vi "Configure Trigger (CAN - Start,EOF,Missing Ack).vi"(0 "VISA resource name":refnum<visa-resource-name>, 1 "Data Threshold (0.0V)":dbl, 2 "Nominal Bit Rate (1MB)":dbl=1000000.0, 3 "CAN Format (0:Standard)":u16(ring) items=["Standard", "Extended"], 5 "Source (0:Channel1)":u16(ring) items=["Channel1", "Channel2", "Channel3", "Channel4"], 7 "Signal Type (0:Differential)":u16(ring) items=["Differential", "CAN + H", "CAN - L", "TX", "RX"], 9 "Trigger Condition (0:Start)":u16(ring) items=["Start"=0, "EOF"=5, "Missing ack"=6], 11 "error in (no error)":errorcluster) -> (4 "VISA resource name out":refnum<visa-resource-name>, 15 "error out":errorcluster)   [LabVIEW 2015, in "Tektronix 7000 Series.lvlib"]
doc: "Configures CAN trigger settings(Start,EOF,Missing Ask) for an oscilloscope.A trigger occurs when a Controller Area Network frame signal is found.\n\n<b>Note:</b>\nOnly DPO7000 series oscilloscopes Support CAN Trigger."
uses:
  <instrlib>/Tektronix 7000 Series/Tektronix 7000 Series.lvlib
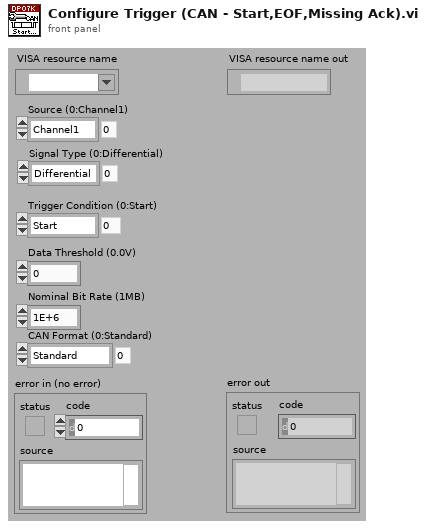
[diagram p1: front panel]
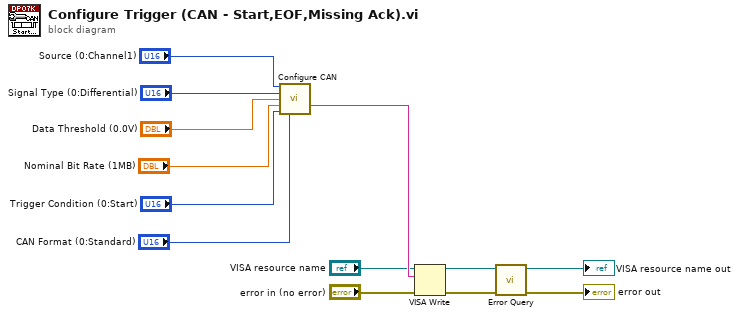
[diagram p0: block diagram]
diagram:
  n1 = call <instrlib>:"Configure CAN.vi"("Source (0:Channel1)"="Source (0:Channel1)", "Signal Type (0:Differential)"="Signal Type (0:Differential)", "Data Threshold (0.0V)"="Data Threshold (0.0V)", "Nominal Bit Rate (1MB)"="Nominal Bit Rate (1MB)", "Trigger Condition (0:Start)"="Trigger Condition (0:Start)", "CAN Format (0:Standard)"="CAN Format (0:Standard)") -> ("Output String"=w11:string)  [unwired: 9 in]
  n2 = VISA Write(VISA resource name="VISA resource name", write buffer=w11, error in (no error)="error in (no error)") -> (VISA resource name out=w12:refnum<visa-resource-name>, error out=w13:errorcluster)  [unwired: 1 out]
  n3 = call <instrlib>:"Error Query.vi"("error in (no error)"=w13, "VISA resource name"=w12) -> ("error out"=→"error out":errorcluster, "VISA resource name out"=→"VISA resource name out":refnum<visa-resource-name>)  [unwired: 6 in, 2 out]
